vi "GitGetHash.vi"(8 "error in (no error)":errorcluster, 9 "Directory":path=path "", 11 "Git exec":string="git") -> (0 "error out":errorcluster, 1 "Directory out":path, 2 "Hash":string, 3 "Git exec out":string="git")   [LabVIEW 2013]
uses:
  GitCmd.vi
  <vilib>/dlg_ctls.llb/Space Constant.vi
  GitUtils/PathtoDirPath.vi
  <vilib>/Platform/system.llb/System Exec.vi
  <vilib>/Utility/error.llb/Error Cluster From Error Code.vi
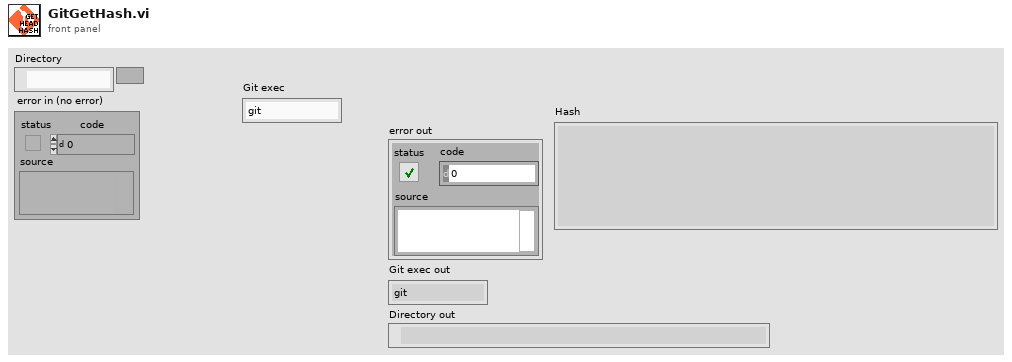
[diagram p1: front panel]
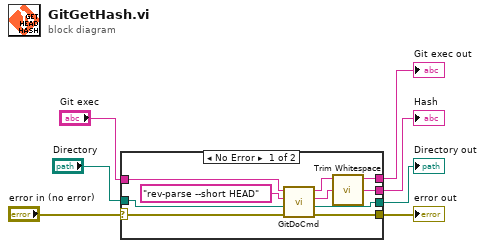
[diagram p0: block diagram]
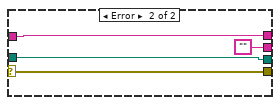
[diagram p2: hidden frame]
diagram:
  n1 = case shown="No Error" "error in (no error)" {
    selector: "error in (no error)" -> [w12 w19]
    tunnel: "Git exec" -> [w8 w17]
    tunnel: "Directory" -> [w11 w18]
    tunnel: [w10 ""] -> w5
    tunnel: [w16 w19] -> w4
    tunnel: [w15 w18] -> w2
    tunnel: [w14 w17] -> w1
    frame No Error {
      n2 = call "GitDoCmd.vi"("error in (no error)"=w12, "Working Path"=w11, "Git command"="rev-parse --short HEAD" ("string"), "Git exec"=w8) -> ("error out"=w16:errorcluster, "Working Path out"=w15:path, "Returned stdout"=w9:string, "Git exec out"=w14:string)  [unwired: 3 in]
      n3 = call <vilib>:"Trim Whitespace.vi"("string"=w9) -> ("trimmed string"=w10:string)  [unwired: 1 in]
    }
    frame Error {
    }
  }
  "Hash" <- w5
  "error out" <- w4
  "Git exec out" <- w1
  "Directory out" <- w2
